vi "UMLEditor_UpdateVI.vi"(1 "ViPath":path, 2 "DependendClasses":refnum<class "AbstractNode.lvclass">[](array[class]), 5 "error in (no error)":errorcluster) -> (19 "error out":errorcluster)   [LabVIEW 2014]
doc: "Gets current diagram values"
uses:
  <resource>/Framework/Providers/Open_GDS/UML/AbstractNode_class/AbstractNode.lvclass
  <resource>/Framework/Providers/Open_GDS/UML/ClassNode_class/ClassNode.lvclass
  <resource>/Framework/Providers/Open_GDS/ClassProviders/Provider_BaseClassInterface/ClassReader_class/ClassReader.lvclass
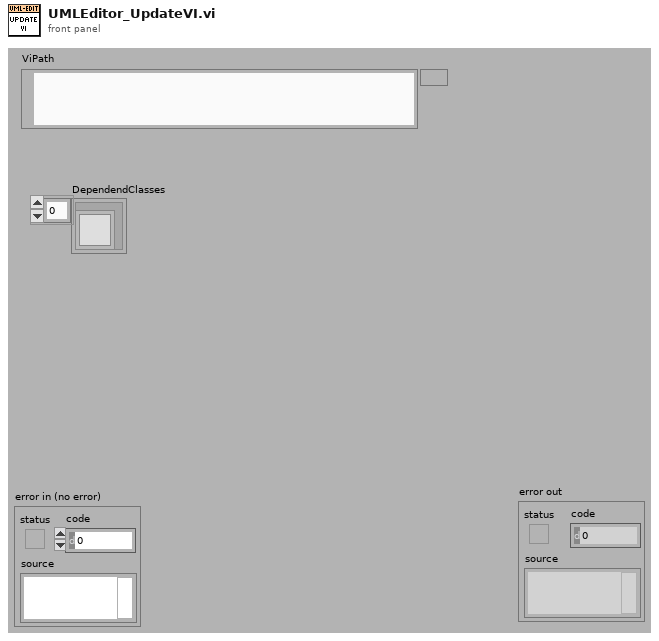
[diagram p1: front panel]
types:
  T1 = cluster{"DepClasses":refnum<class "ClassNode.lvclass">[], "ClassPathes":path[], "ClassesPublicVIs":cluster{"PublicVIs":path[]}[], "StartPos":cluster{i32, u32}, "BD":refnum<vi>, "ViRef":refnum<vi>}
  T2 = typedef "ClassTypes_MethodType.ctl" = cluster{"MethodName":string, "Visibility":enum16{"Public", "Private", "Protected"}, "StereoType":string, "Path":path}
  T3 = typedef "Librarian File Info Out.ctl" = cluster{"creation date":u32, "last mod date":u32, "type":string, "creator":string, "LV version":i32, "size":i32, "top level":bool}
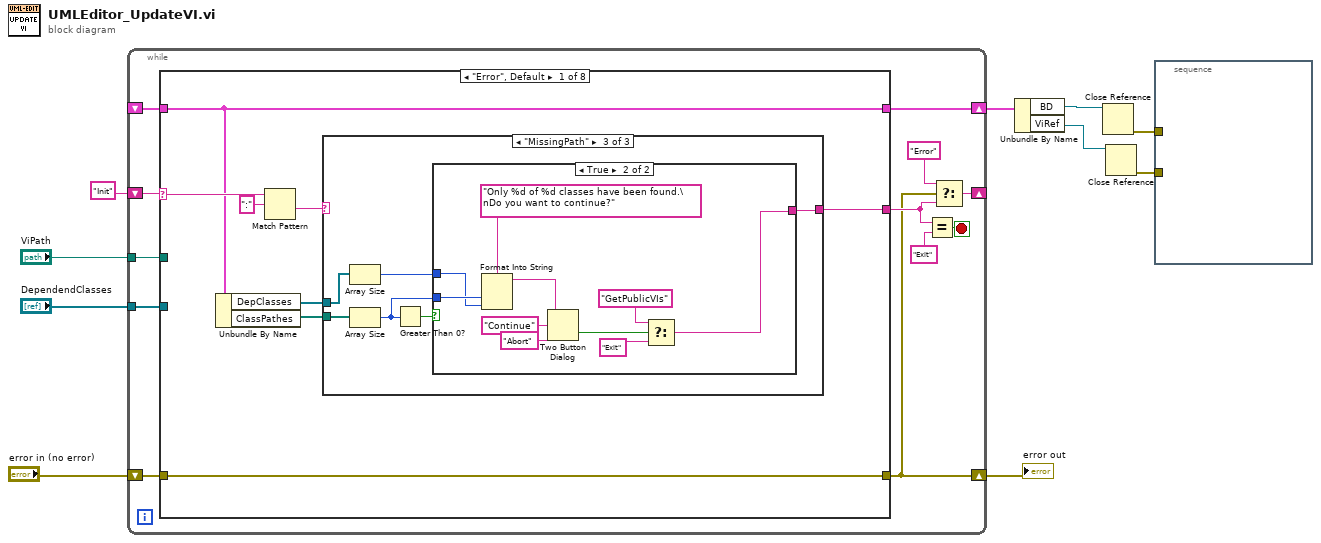
[diagram p0: block diagram]
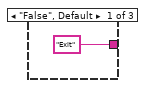
[diagram p2: hidden frame]
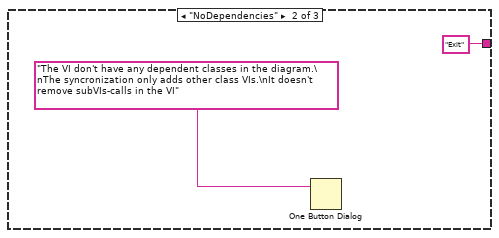
[diagram p3: hidden frame]
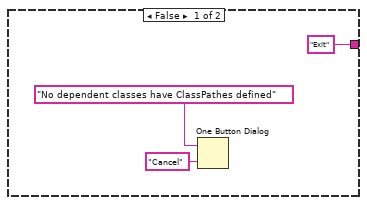
[diagram p4: hidden frame]
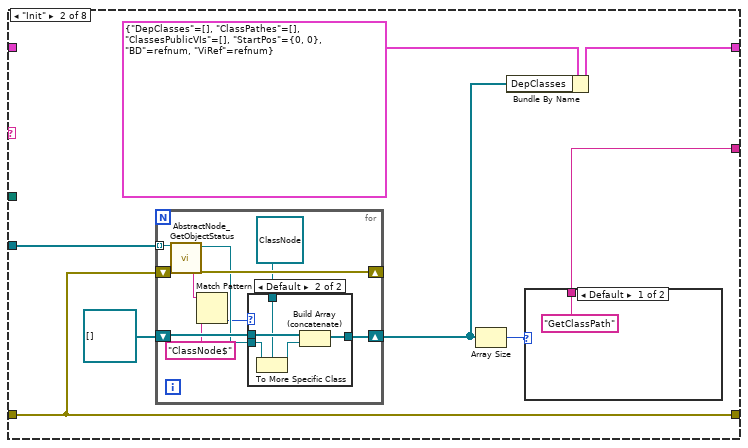
[diagram p5: hidden frame]
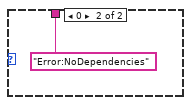
[diagram p6: hidden frame]
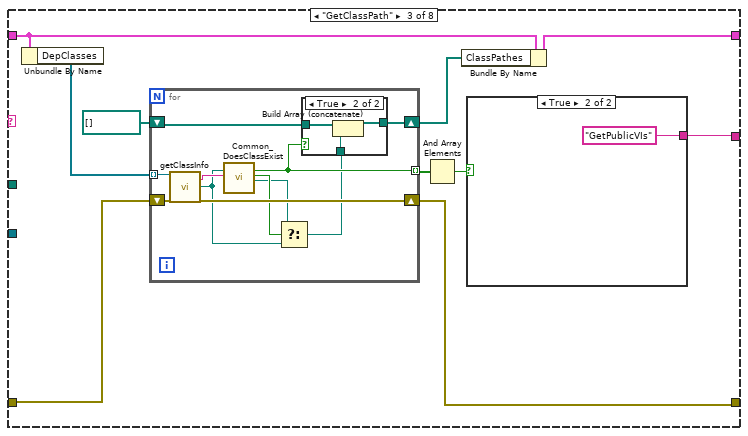
[diagram p8: hidden frame]
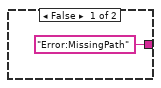
[diagram p9: hidden frame]
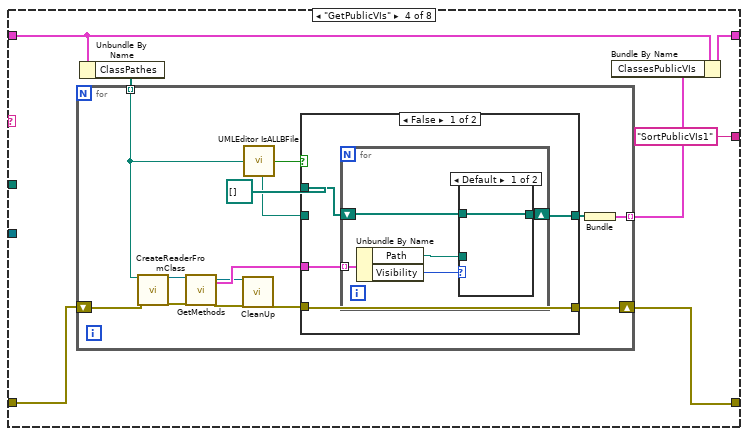
[diagram p11: hidden frame]
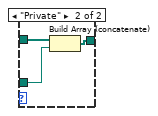
[diagram p12: hidden frame]
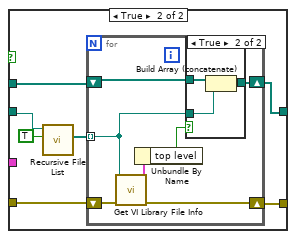
[diagram p13: hidden frame]
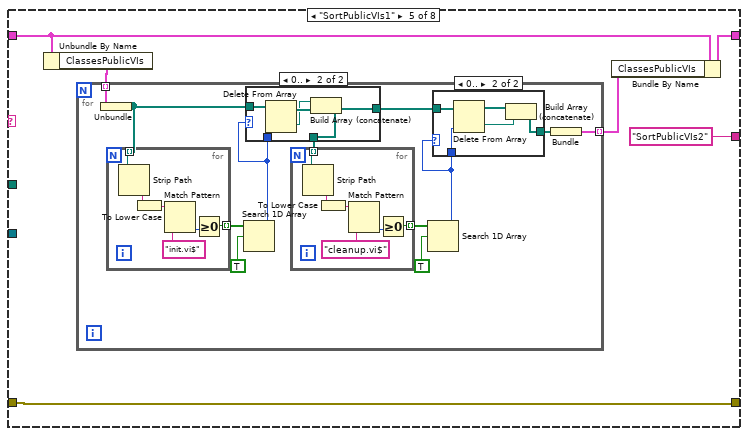
[diagram p15: hidden frame]
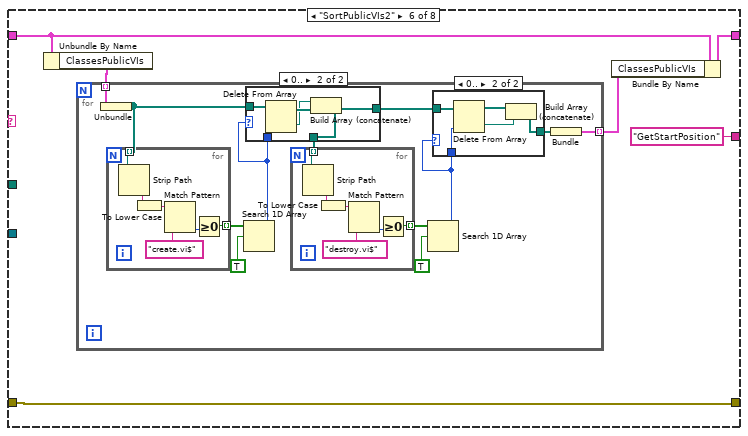
[diagram p18: hidden frame]
diagram:
  n1 = while {
    shift-right: [w15] -> w8
    shift-left: "error in (no error)" -> [w22]
    shift-right: [w20] -> _
    shift-left: "Init" -> [w21]
    shift-right: [w14] -> w5
    shift-left: _ -> [w13]
    tunnel: "ViPath" -> [w11]
    tunnel: "DependendClasses" -> [w12]
    stop <- w19 stop-if-true
    n2 = case shown="\"Error\", Default" w21 {
      selector: w21 -> [w29 _ _ _ _ _ _ _]
      tunnel: w22 -> [w30 w59 w87 w111 w158 w200 w241 w277]
      tunnel: [w30 w59 w79 w107 w158 w200 w255 w278] -> w15
      tunnel: [w24 w54 w80 "SortPublicVIs1" "SortPublicVIs2" "GetStartPosition" "PlaceMethodsOnDiagram" "Exit"] -> w16
      tunnel: [w26 w56 w83 w109 w160 w202 w257 w273] -> w14
      tunnel: w13 -> [w26 _ w84 w110 w161 w203 w259 w273]
      tunnel: w12 -> [_ w60 _ _ _ _ _ _]
      tunnel: w11 -> [_ _ _ _ _ _ w242 _]
      frame "Error", Default {
        n3 = Unbundle By Name(w26) -> ("DepClasses"=w23:refnum<class "ClassNode.lvclass">[], "ClassPathes"=w25:path[])
        n4 = Match Pattern(string=w29, regular expression=":") -> (after substring=w27:string)  [unwired: 4 out]
        n5 = case shown="\"MissingPath\"" w27 {
          tunnel: w25 -> [_ _ w39]
          tunnel: ["Exit" "Exit" w37] -> w24
          tunnel: w23 -> [_ _ w35]
          frame "False", Default {
          }
          frame "NoDependencies" {
            n6 = One Button Dialog(message="The VI don't have any dependent classes in the diagram.\nThe syncronization only adds other class VIs.\nIt doesn't remove subVIs-calls in the VI") -> ()  [unwired: 2 out]
          }
          frame "MissingPath" {
            n7 = Array Size(array=w35) -> (size(s)=w34:i32)
            n8 = Array Size(array=w39) -> (size(s)=w36:i32)
            n9 = Greater Than 0?(x=w36) -> (x > 0?=w38:bool)
            n10 = case shown="True" w38 {
              tunnel: ["Exit" w43] -> w37
              tunnel: w36 -> [_ w52]
              tunnel: w34 -> [_ w51]
              frame False {
                n11 = One Button Dialog(message="No dependent classes have ClassPathes defined", button name ("OK")="Cancel") -> ()  [unwired: 1 out]
              }
              frame True {
                n12 = Format Into String(format string="Only %d of %d classes have been found.\nDo you want to continue?" ("message"), w52, w51) -> (resulting string=w49:string)  [unwired: 2 in, 1 out]
                n13 = Two Button Dialog(message=w49, 1:"Abort" ("F button name (\"Cancel\")"), 2:"Continue" ("T button name (\"OK\")")) -> (T button?=w46:bool)
                n14 = Select(t="GetPublicVIs", s=w46, f="Exit") -> (s? t:f=w43:string)
              }
            }
          }
        }
      }
      frame "Init" {
        n15 = for {
          shift-right: [w70] -> _
          shift-left: w59 -> [w72]
          tunnel: w60 -> [w71] mode=indexing
          shift-right: [w67] -> w53
          shift-left: refnum<class "ClassNode.lvclass">[] [] -> [w69]
          n16 = call <resource>:"AbstractNode_GetObjectStatus.vi"("reference in"=w71, "error in (no error)"=w72) -> ("Class name"=w66:string, "reference out"=w68:refnum<class "AbstractNode.lvclass">, "error out"=w70:errorcluster)  [unwired: 15 out]
          n17 = Match Pattern(string=w66, regular expression="ClassNode$") -> (offset past match=w64:i32)  [unwired: 4 out]
          n18 = case shown="Default" w64 {
            tunnel: w69 -> [w73 w78]
            tunnel: w68 -> [_ w76]
            tunnel: [w73 w77] -> w67
            tunnel: refnum<class "ClassNode.lvclass"> refnum ("reference") -> [_ w74]
            frame -1 {
            }
            frame Default {
              n19 = To More Specific Class(target class=w74, reference=w76) -> (specific class reference=w75:refnum<class "ClassNode.lvclass">)  [unwired: 1 in, 1 out]
              n20 = Build Array (concatenate)(w78, w75) -> (w77:refnum<class "ClassNode.lvclass">[])
            }
          }
        }
        n21 = Array Size(array=w53) -> (size(s)=w55:i32)
        n22 = Bundle By Name(cluster=T1 {"DepClasses"=[], "ClassPathes"=[], "ClassesPublicVIs"=[], "StartPos"={0, 0}, "BD"=refnum, "ViRef"=refnum}, "DepClasses"=w53) -> (w56:T1)
        n23 = case shown="Default" w55 {
          tunnel: ["GetClassPath" "Error:NoDependencies"] -> w54
          frame Default {
          }
          frame 0 {
          }
        }
      }
      frame "GetClassPath" {
        n24 = Unbundle By Name(w84) -> ("DepClasses"=w88:refnum<class "ClassNode.lvclass">[])
        n25 = for {
          tunnel: w88 -> [w91] mode=indexing
          shift-right: [w100] -> w79
          shift-left: w87 -> [w101]
          tunnel: [w98] -> w86 mode=indexing
          shift-right: [w96] -> w81
          shift-left: path[] [] -> [w97]
          n26 = call-dynamic "getClassInfo.vi"("reference"=w91, "error in (no error)"=w101) -> ("className"=w99:string, "ClassPath"=w93:path, "error out"=w100:errorcluster)  [unwired: 8 in, 7 out]
          n27 = call <resource>:"Common_DoesClassExist.vi"("ClassPath"=w93, "ClassName"=w99) -> ("ClassExists"=w98:bool, "llb-class"=w95:bool, "llb/LvCLass-Path"=w94:path)  [unwired: 15 out]
          n28 = Select(t=w94, s=w95, f=w93) -> (s? t:f=w92:path)
          n29 = case shown="True" w98 {
            tunnel: w97 -> [w102 w105]
            tunnel: [w102 w104] -> w96
            tunnel: w92 -> [_ w103]
            frame False {
            }
            frame True {
              n30 = Build Array (concatenate)(w105, w103) -> (w104:path[])
            }
          }
        }
        n31 = And Array Elements(Boolean array=w86) -> (logical AND=w85:bool)
        n32 = Bundle By Name(cluster=w84, "ClassPathes"=w81) -> (w83:T1)
        n33 = case shown="True" w85 {
          tunnel: ["Error:MissingPath" "GetPublicVIs"] -> w80
          frame False {
          }
          frame True {
          }
        }
      }
      frame "GetPublicVIs" {
        n34 = Unbundle By Name(w110) -> ("ClassPathes"=w112:path[])
        n35 = for {
          tunnel: w112 -> [w117] mode=indexing
          shift-right: [w121] -> w107
          shift-left: w111 -> [w120]
          tunnel: [w123] -> w108 mode=indexing
          n36 = call <resource>:"CreateReaderFromClass.vi"("ClassPath/LvClassRef"=w117, "error in"=w120) -> ("ClassReader"=w119:refnum<class "ClassReader.lvclass">, "error out"=w118:errorcluster)  [unwired: 16 out]
          n37 = call-dynamic "GetMethods.vi"("ClassReader in"=w119, "error in (no error)"=w118) -> ("ClassReader out"=w115:refnum<class "ClassReader.lvclass">, "Methods"=w116:T2[], "error out"=w114:errorcluster)  [unwired: 15 out]
          n38 = call-dynamic "CleanUp.vi"("reference in"=w115, "error in (no error)"=w114) -> ("error out"=w113:errorcluster)  [unwired: 17 out]
          n39 = call <resource>:"UMLEditor IsALLBFile.vi"("path"=w117) -> ("path to VI library?"=w125:bool)
          n40 = case shown="False" w125 {
            tunnel: w113 -> [w129 w145]
            tunnel: w117 -> [_ w141]
            tunnel: [w128 w143] -> w124
            tunnel: path[] [] -> [w127 w144]
            tunnel: [w129 w142] -> w121
            tunnel: w116 -> [w126 _]
            frame False {
              n41 = for {
                shift-right: [w134] -> w128
                shift-left: w127 -> [w133]
                tunnel: w126 -> [w132] mode=indexing
                n42 = Unbundle By Name(w132) -> ("Path"=w130:path, "Visibility"=w131:enum16{"Public", "Private", "Protected"})
                n43 = case shown="Default" w131 {
                  tunnel: [w135 w138] -> w134
                  tunnel: w133 -> [w135 w137]
                  tunnel: w130 -> [_ w136]
                  frame Default {
                  }
                  frame "Private" {
                    n44 = Build Array (concatenate)(w137, w136) -> (w138:path[])
                  }
                }
              }
            }
            frame True {
              n45 = call <vilib>:"Recursive File List.vi"("Treat LLBs as Folders?"=TRUE, "Folder Path"=w141) -> ("All Files in Dir"=w139:path[])  [unwired: 1 in, 8 out]
              n46 = for {
                shift-right: [w150] -> w142
                shift-left: w145 -> [w151]
                shift-right: [w147] -> w143
                shift-left: w144 -> [w148]
                tunnel: w139 -> [w146] mode=indexing
                n47 = call <vilib>:"Get VI Library File Info.vi"("error in (no error)"=w151, "path"=w146) -> ("error out"=w150:errorcluster, "file information"=w152:T3)  [unwired: 8 out]
                n48 = Unbundle By Name(w152) -> ("top level"=w149:bool)
                n49 = case shown="True" w149 {
                  tunnel: w148 -> [w153 w156]
                  tunnel: [w153 w155] -> w147
                  tunnel: w146 -> [_ w154]
                  frame False {
                  }
                  frame True {
                    n50 = Build Array (concatenate)(w156, w154) -> (w155:path[])
                  }
                }
              }
            }
          }
          n51 = Bundle(w124) -> (w123:cluster{path[]})  [unwired: 1 in]
        }
        n52 = Bundle By Name(cluster=w110, "ClassesPublicVIs"=w108) -> (w109:T1)
      }
      frame "SortPublicVIs1" {
        n53 = Unbundle By Name(w161) -> ("ClassesPublicVIs"=w162:cluster{"PublicVIs":path[]}[])
        n54 = for {
          tunnel: w162 -> [w174] mode=indexing
          tunnel: [w173] -> w157 mode=indexing
          n55 = Unbundle(w174) -> ("PublicVIs"=w170:path[])
          n56 = for {
            tunnel: w170 -> [w198] mode=indexing
            tunnel: [w193] -> w172 mode=indexing
            n57 = Strip Path(path=w198) -> (name=w196:string)  [unwired: 1 out]
            n58 = To Lower Case(string=w196) -> (all lower case string=w197:string)
            n59 = Match Pattern(string=w197, regular expression="init.vi$") -> (offset past match=w194:i32)  [unwired: 4 out]
            n60 = Greater Or Equal To 0?(x=w194) -> (x >= 0?=w193:bool)
          }
          n61 = Search 1D Array(1D array=w172, element=TRUE) -> (index of element=w165:i32)  [unwired: 1 out]
          n62 = case shown="0.." w165 {
            tunnel: w170 -> [w181 w186]
            tunnel: w165 -> [_ w185]
            tunnel: [w181 w182] -> w167
            tunnel: [w181 w182] -> w164
            frame -1, Default {
            }
            frame 0.. {
              n63 = Delete From Array(array=w186, index=w185) -> (deleted portion=w183:path, array with subset deleted=w184:path[])  [unwired: 1 in]
              n64 = Build Array (concatenate)(w183, w184) -> (w182:path[])
            }
          }
          n65 = for {
            tunnel: w167 -> [w192] mode=indexing
            tunnel: [w187] -> w168 mode=indexing
            n66 = Strip Path(path=w192) -> (name=w190:string)  [unwired: 1 out]
            n67 = To Lower Case(string=w190) -> (all lower case string=w191:string)
            n68 = Match Pattern(string=w191, regular expression="cleanup.vi$") -> (offset past match=w188:i32)  [unwired: 4 out]
            n69 = Greater Or Equal To 0?(x=w188) -> (x >= 0?=w187:bool)
          }
          n70 = Search 1D Array(1D array=w168, element=TRUE) -> (index of element=w163:i32)  [unwired: 1 out]
          n71 = case shown="0.." w163 {
            tunnel: w163 -> [_ w180]
            tunnel: [w175 w177] -> w166
            tunnel: w164 -> [w175 w176]
            frame -1, Default {
            }
            frame 0.. {
              n72 = Delete From Array(array=w176, index=w180) -> (deleted portion=w178:path, array with subset deleted=w179:path[])  [unwired: 1 in]
              n73 = Build Array (concatenate)(w179, w178) -> (w177:path[])
            }
          }
          n74 = Bundle("PublicVIs"=w166) -> (w173:cluster{"PublicVIs":path[]})  [unwired: 1 in]
        }
        n75 = Bundle By Name(cluster=w161, "ClassesPublicVIs"=w157) -> (w160:T1)
      }
      frame "SortPublicVIs2" {
        n76 = Unbundle By Name(w203) -> ("ClassesPublicVIs"=w204:cluster{"PublicVIs":path[]}[])
        n77 = for {
          tunnel: w204 -> [w216] mode=indexing
          tunnel: [w215] -> w199 mode=indexing
          n78 = Unbundle(w216) -> ("PublicVIs"=w212:path[])
          n79 = for {
            tunnel: w212 -> [w240] mode=indexing
            tunnel: [w235] -> w214 mode=indexing
            n80 = Strip Path(path=w240) -> (name=w238:string)  [unwired: 1 out]
            n81 = To Lower Case(string=w238) -> (all lower case string=w239:string)
            n82 = Match Pattern(string=w239, regular expression="create.vi$") -> (offset past match=w236:i32)  [unwired: 4 out]
            n83 = Greater Or Equal To 0?(x=w236) -> (x >= 0?=w235:bool)
          }
          n84 = Search 1D Array(1D array=w214, element=TRUE) -> (index of element=w207:i32)  [unwired: 1 out]
          n85 = case shown="0.." w207 {
            tunnel: w212 -> [w223 w228]
            tunnel: w207 -> [_ w227]
            tunnel: [w223 w224] -> w209
            tunnel: [w223 w224] -> w206
            frame -1, Default {
            }
            frame 0.. {
              n86 = Delete From Array(array=w228, index=w227) -> (deleted portion=w225:path, array with subset deleted=w226:path[])  [unwired: 1 in]
              n87 = Build Array (concatenate)(w225, w226) -> (w224:path[])
            }
          }
          n88 = for {
            tunnel: w209 -> [w234] mode=indexing
            tunnel: [w229] -> w210 mode=indexing
            n89 = Strip Path(path=w234) -> (name=w232:string)  [unwired: 1 out]
            n90 = To Lower Case(string=w232) -> (all lower case string=w233:string)
            n91 = Match Pattern(string=w233, regular expression="destroy.vi$") -> (offset past match=w230:i32)  [unwired: 4 out]
            n92 = Greater Or Equal To 0?(x=w230) -> (x >= 0?=w229:bool)
          }
          n93 = Search 1D Array(1D array=w210, element=TRUE) -> (index of element=w205:i32)  [unwired: 1 out]
          n94 = case shown="0.." w205 {
            tunnel: w205 -> [_ w222]
            tunnel: [w217 w219] -> w208
            tunnel: w206 -> [w217 w218]
            frame -1, Default {
            }
            frame 0.. {
              n95 = Delete From Array(array=w218, index=w222) -> (deleted portion=w220:path, array with subset deleted=w221:path[])  [unwired: 1 in]
              n96 = Build Array (concatenate)(w221, w220) -> (w219:path[])
            }
          }
          n97 = Bundle("PublicVIs"=w208) -> (w215:cluster{"PublicVIs":path[]})  [unwired: 1 in]
        }
        n98 = Bundle By Name(cluster=w203, "ClassesPublicVIs"=w199) -> (w202:T1)
      }
      frame "GetStartPosition" {
        n99 = call <resource>:"CommonVIs_UmlOpenVIRef.vi"("error in"=w241, "ViPath/ViName"=w242) -> ("error out"=w244:errorcluster, "vi reference"=w243:refnum<vi>)  [unwired: 2 in, 6 out]
        n100 = property class="VI"(reference=w243, error in=w244, "Front Panel Window:Open"=TRUE) -> (reference out=w247:refnum<vi>, error out=w245:errorcluster, "Block Diagram"=w252:refnum<vi>)
        n101 = property class="TopLvlDiag"(reference=w252, error in=w245, "Selected"=FALSE, "Position"=cluster{"Left":i32, "Top":i32} {"Left"=0, "Top"=0}) -> (reference out=w248:refnum<vi>, error out=w246:errorcluster)
        n102 = property class="TopLvlDiag"(reference=w248, error in=w246) -> (reference out=w254:refnum<vi>, error out=w255:errorcluster, "All Objects[]"=w265:refnum<vi>[])
        n103 = for {
          tunnel: w265 -> [w272] mode=indexing
          tunnel: [w269] -> w264 mode=indexing
          tunnel: [w268] -> w263 mode=indexing
          tunnel: [w266] -> _
          n104 = property class="GObj"(reference=w272) -> (reference out=w267:refnum<vi>, "Position:Left"=w269:i32, "Position:Top"=w271:i32, "Bounds:Height"=w270:u32)  [unwired: 1 in, 1 out]
          n105 = Add(x=w271, y=w270) -> (x+y=w268:u32)
          n106 = Close Reference(reference=w267) -> (error out=w266:errorcluster)  [unwired: 1 in]
        }
        n107 = Array Max & Min(array=w264) -> (min value=w249:i32)  [unwired: 3 out]
        n108 = Array Max & Min(array=w263) -> (max value=w262:u32)  [unwired: 3 out]
        n109 = Add(x=w262, y=u32 16) -> (x+y=w260:u32)
        n110 = Bundle(w249, w260) -> (w258:cluster{i32, u32})  [unwired: 1 out]
        n111 = Bundle By Name(cluster=w259, "ViRef"=w247, "BD"=w254, "StartPos"=w258) -> (w257:T1)
      }
      frame "PlaceMethodsOnDiagram" {
        n112 = Unbundle By Name(w273) -> ("BD"=w275:refnum<vi>, "StartPos"=w276:cluster{i32, u32}, "ClassesPublicVIs"=w279:cluster{"PublicVIs":path[]}[])
        n113 = for {
          tunnel: w279 -> [w287] mode=indexing
          shift-right: [w280] -> w278
          shift-left: w277 -> [w286]
          shift-right: [w281] -> _
          shift-left: w276 -> [w283]
          tunnel: w275 -> [w284]
          n114 = Unbundle(w287) -> ("PublicVIs"=w285:path[])
          n115 = call <resource>:"UMLEditor_PlaceVIsOnBlockDiagram.vi"("BD"=w284, "StartPos"=w283, "VIs"=w285, "error in (no error)"=w286) -> ("error out"=w280:errorcluster)  [unwired: 15 out]
          n116 = Add(x=w283, y=cluster{i32, u32} {0, 64}) -> (x+y=w281:cluster{i32, u32})
        }
      }
    }
    n117 = Equal?(x=w16, y="Exit") -> (x = y?=w19:bool)
    n118 = Select(t="Error", s=w15, f=w16) -> (s? t:f=w20:string)
  }
  "error out" <- w8
  n119 = Unbundle By Name(w5) -> ("BD"=w4:refnum<vi>, "ViRef"=w3:refnum<vi>)
  n120 = Close Reference(reference=w4) -> (error out=w2:errorcluster)  [unwired: 1 in]
  n121 = Close Reference(reference=w3) -> (error out=w1:errorcluster)  [unwired: 1 in]
  n122 = stacked-sequence {
    tunnel: w2 -> [_]
    tunnel: w1 -> [_]
    frame #0 {
    }
  }
